vi "Set analog voltage on slow analog output.vi"() -> ()   [LabVIEW 2010]
doc: "This example shows how to set analog voltage of slow analog outputs on Red Pitaya extension connector. Slow analog outputs on Red Pitaya are in range from 0 to 1.8 Volts."
uses:
  RedPitaya.lvlib
panel:
  in  "Analog Voltage Value":dbl=1.34
  in  "Pin #":u16(ring)=3 items=["AOUT0", "AOUT1", "AOUT2", "AOUT3"]
  in  "IP address":string="192.168.4.129"
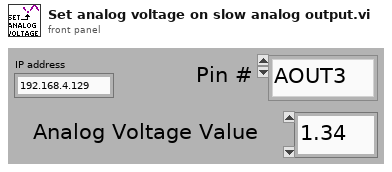
[diagram p1: front panel]
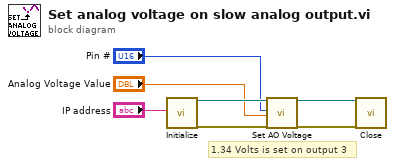
[diagram p0: block diagram]
diagram:
  # "1.34 Volts is set on output 3"
  n1 = call "Initialize.vi"("IP address"="IP address") -> ("RedPitaya TCP Connection"=w6:refnum<k5>, "error out"=w5:errorcluster)  [unwired: 17 in]
  n2 = call "Set AO Voltage.vi"("RedPitaya connection in"=w6, "Pin #"="Pin #", "Analog Voltage Value"="Analog Voltage Value", "error in"=w5) -> ("RedPitaya connection out"=w3:refnum<k5>, "error out"=w4:errorcluster)  [unwired: 14 in]
  n3 = call "Close.vi"("connection ID"=w3, "error in"=w4) -> ()  [unwired: 17 in, 1 out]
